vi "checkPython.vi"() -> ()   [LabVIEW 2015]
panel:
  out "status_bar":string="Finalize\nCosmedAPTools installation....."
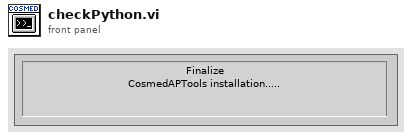
[diagram p1: front panel]
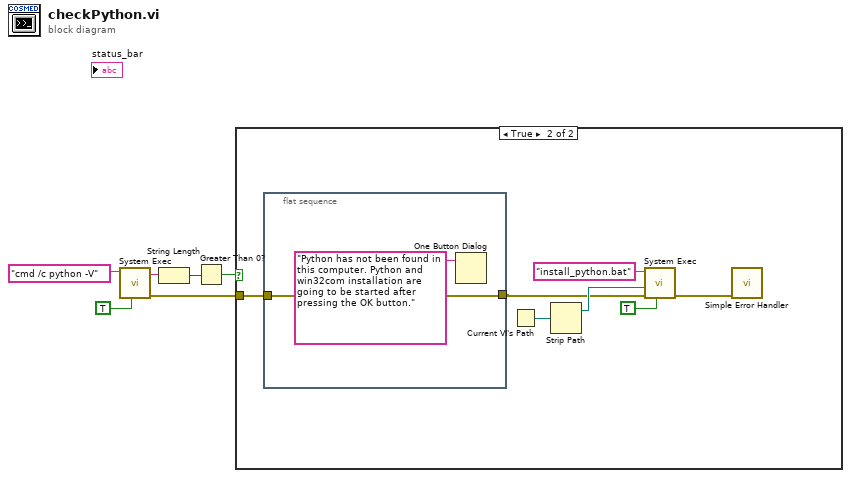
[diagram p0: block diagram]
diagram:
  n1 = call <vilib>:"System Exec.vi"("run minimized? (F)"=TRUE, "command line"="cmd /c python -V") -> ("error out"=w1:errorcluster, "standard output"=w5:string)  [unwired: 4 in, 4 out]
  n2 = String Length(string=w5) -> (length=w4:i32)
  n3 = Greater Than 0?(x=w4) -> (x > 0?=w2:bool)
  n4 = case shown="True" w2 {
    tunnel: w1 -> [_ w13]
    frame False {
    }
    frame True {
      n5 = flat-sequence {
        tunnel: w13 -> [w14]
        tunnel: [w14] -> w9
        frame #0 {
          n6 = One Button Dialog(message="Python has not been found in this computer. Python and win32com installation are going to be started after pressing the OK button.") -> ()  [unwired: 1 in, 1 out]
        }
      }
      n7 = Current VI's Path() -> (path=w11:path)
      n8 = Strip Path(path=w11) -> (stripped path=w10:path)  [unwired: 1 out]
      n9 = call <vilib>:"System Exec.vi"("run minimized? (F)"=TRUE, "error in (no error)"=w9, "working directory"=w10, "command line"="install_python.bat") -> ("error out"=w8:errorcluster)  [unwired: 2 in, 5 out]
      n10 = call <vilib>:"Simple Error Handler.vi"("error in (no error)"=w8) -> ()  [unwired: 4 in, 5 out]
    }
  }
